vi "FTW-Container-Element-SetContainer.vi"(0 "FTW-Container In":refnum<class "FTW-Container.lvclass">, 5 "Element Name":string, 7 "Value":refnum<class "FTW-Container.lvclass">, 11 "error in":errorcluster) -> (4 "FTW-Container Out":refnum<class "FTW-Container.lvclass">, 8 "Replaced":bool, 15 "error out":errorcluster)   [LabVIEW 2015, in "FTW-Container.lvclass"]
uses:
  FTW-Container.lvclass
  FTW-Container.lvclass/FTW-Container.ctl
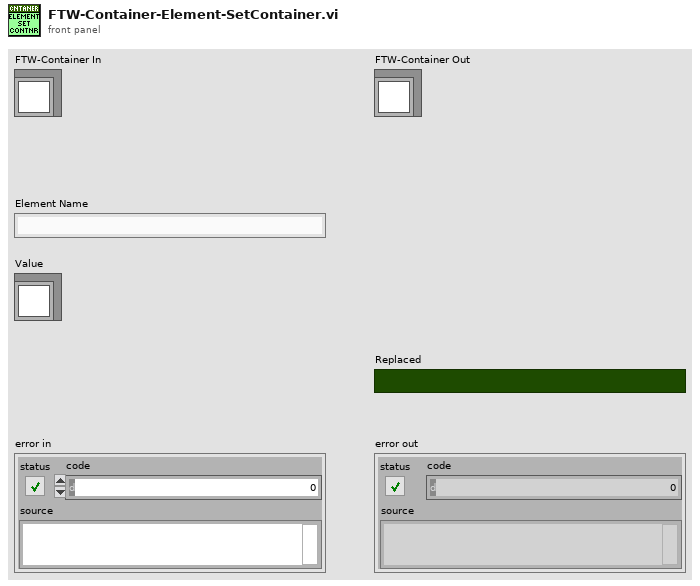
[diagram p1: front panel]
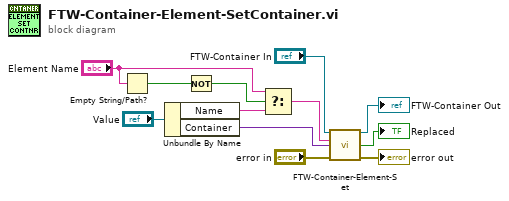
[diagram p0: block diagram]
diagram:
  n1 = Empty String/Path?(string/path="Element Name") -> (empty?=w5:bool)
  n2 = Unbundle By Name("Value") -> ("Name"=w2:string, "Container"=w6:variant)
  n3 = Not(x=w5) -> (.not. x?=w4:bool)
  n4 = Select(t="Element Name", s=w4, f=w2) -> (s? t:f=w1:string)
  n5 = call "FTW-Container-Element-Set.vi"("FTW-Container In"="FTW-Container In", "Element Name"=w1, "Value"=w6, "error in"="error in") -> ("FTW-Container Out"=→"FTW-Container Out":refnum<class "FTW-Container.lvclass">, "Replaced"=→"Replaced":bool, "error out"=→"error out":errorcluster)  [unwired: 9 in]
